vi "4.Dashboard.vi"() -> ()   [LabVIEW 2023]
uses:
  UnderAutomation.UniversalRobots.lvlib
panel:
  out "Boolean":bool=TRUE
  in  "OK Button":bool
  in  "stop":bool
  out "Response":cluster{"Message":string, "Succeed":bool}
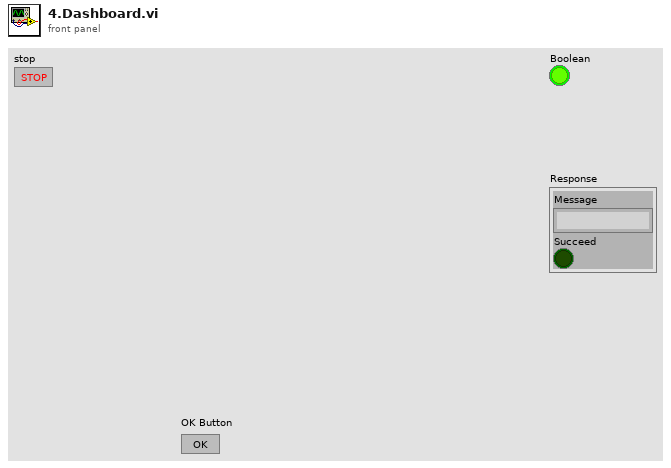
[diagram p1: front panel]
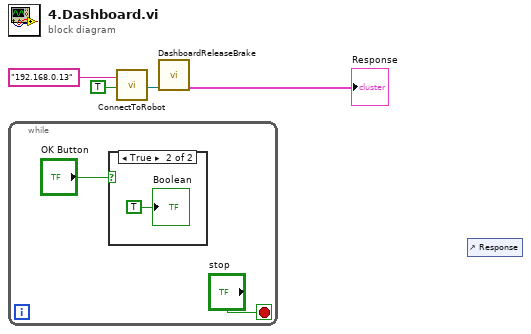
[diagram p0: block diagram]
diagram:
  n1 = while {
    stop <- "stop" stop-if-true
    n2 = case shown="True" "OK Button" {
      frame False {
      }
      frame True {
        "Boolean" <- TRUE
      }
    }
  }
  n3 = call "ConnectToRobot.vi"("ip"="192.168.0.13", "Enable Dashboard"=TRUE) -> ("Dashboard"=w2:refnum<k24>)  [unwired: 13 in, 4 out]
  n4 = call "DashboardReleaseBrake.vi"("Dashboard"=w2) -> ("Response"=→"Response":cluster{"Message":string, "Succeed":bool})  [unwired: 9 in, 1 out]
  n5 = control-ref of="Response"() -> ()  [unwired: 1 out]
